vi "readFromXML.vi"(8 "error in (no error)":errorcluster, 10 "XML in":string, 11 "ProperMotion in":refnum<class "ProperMotion.lvclass">) -> (0 "error out":errorcluster, 3 "ProperMotion out":refnum<class "ProperMotion.lvclass">)   [LabVIEW 2022 SP3, in "TCSDataDefinitions.lvlib" / "TCSCommand.lvlib" / "TargetConfiguration.lvlib" / "Target.lvlib" / "FixedTarget.lvlib" / "ProperMotion.lvclass"]
uses:
  ProperMotion.lvclass
  <userlib>/Common/UnitsAndXML/FlattenItemWithUnitToXML/FlattenAngularVelocityToXML/AngularVelocityUnit.ctl
  ProperMotion.lvclass/ProperMotion.ctl
  <userlib>/Common/UnitsAndXML/UnitsAndXML.lvlib
  <userlib>/Common/XML/XMLParser/XMLParser.lvclass
panel:
  out "pmra_SPYr":dbl
  out "pmdec_ArcsPYr":dbl[unit]
  out "epochPM_Yr":dbl
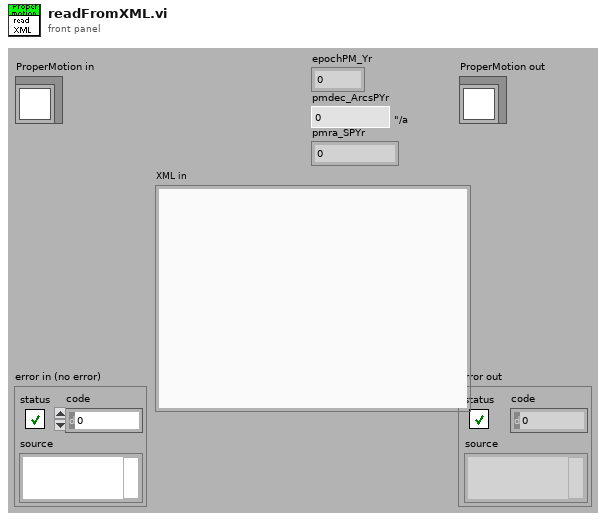
[diagram p1: front panel]
types:
  T1 = typedef "UnitsAndXML.lvlib/AngularVelocityUnit.ctl" = enum16{"\"/a", "deg/s", "\"/s"}
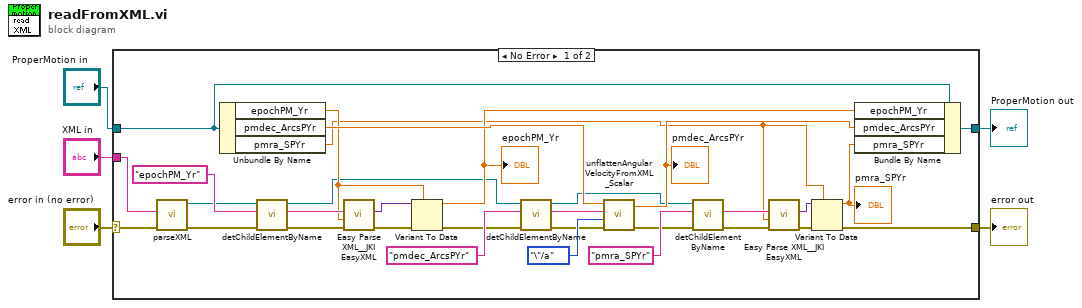
[diagram p0: block diagram]
diagram:
  n1 = case shown="No Error" "error in (no error)" {
    selector: "error in (no error)" -> [w34 w38]
    tunnel: [w12 w38] -> w4
    tunnel: [w27 w37] -> w2
    tunnel: "ProperMotion in" -> [w28 w37]
    tunnel: "XML in" -> [w36 _]
    frame No Error {
      n2 = call <userlib>:"parseXML.vi"("error in (no error)"=w34, "XMLString in"=w36) -> ("error out"=w35:errorcluster, "Element out"=w8:refnum<class "XMLParser.lvclass">)  [unwired: 8 in]
      n3 = Unbundle By Name(w28) -> ("epochPM_Yr"=w19:dbl, "pmdec_ArcsPYr"=w26:dbl[unit], "pmra_SPYr"=w10:dbl[unit])
      n4 = call <userlib>:"detChildElementByName.vi"("error in (no error)"=w35, "childName"="epochPM_Yr" ("ChildName"), "Element in"=w8) -> ("error out"=w21:errorcluster, "childXML"=w20:string, "Element out"=w7:refnum<class "XMLParser.lvclass">)  [unwired: 5 in, 1 out]
      n5 = call <vilib>:"Easy Parse XML__JKI EasyXML.vi"("error in (no error)"=w21, "LabVIEW Data (Type)"=w19, "XML String"=w20) -> ("error out"=w30:errorcluster, "LabVIEW Data"=w29:variant)  [unwired: 7 in]
      n6 = Variant To Data(error in=w30, type=w19, Variant=w29) -> (data=w18:dbl, error out=w9:errorcluster)
      "epochPM_Yr" <- w18
      n7 = call <userlib>:"detChildElementByName.vi"("error in (no error)"=w9, "childName"="pmdec_ArcsPYr" ("ChildName"), "Element in"=w7) -> ("error out"=w23:errorcluster, "childXML"=w25:string, "Element out"=w6:refnum<class "XMLParser.lvclass">)  [unwired: 5 in, 1 out]
      n8 = call <userlib>:"unflattenAngularVelocityFromXML_Scalar.vi"("error in (no error)"=w23, "angularVelocityUnitInXML"=AngularVelocityUnit."\"/a", "xmlString"=w25, "angularVelocityForType"=w26) -> ("error out"=w22:errorcluster, "angularVelocity"=w17:dbl[unit])  [unwired: 6 in]
      "pmdec_ArcsPYr" <- w17
      n9 = call <userlib>:"detChildElementByName.vi"("error in (no error)"=w22, "childName"="pmra_SPYr" ("ChildName"), "Element in"=w6) -> ("error out"=w13:errorcluster, "childXML"=w14:string)  [unwired: 5 in, 2 out]
      n10 = call <vilib>:"Easy Parse XML__JKI EasyXML.vi"("error in (no error)"=w13, "LabVIEW Data (Type)"=w10, "XML String"=w14) -> ("error out"=w16:errorcluster, "LabVIEW Data"=w15:variant)  [unwired: 7 in]
      n11 = Variant To Data(error in=w16, type=w10, Variant=w15) -> (data=w11:dbl[unit], error out=w12:errorcluster)
      "pmra_SPYr" <- w11
      n12 = Bundle By Name(cluster=w28, "epochPM_Yr"=w18, "pmdec_ArcsPYr"=w17, "pmra_SPYr"=w11) -> (w27:refnum<class "ProperMotion.lvclass">)
    }
    frame Error {
    }
  }
  "error out" <- w4
  "ProperMotion out" <- w2
